vi "test Initial Label.vi"(8 "error in (no error)":errorcluster, 11 "TestCase in":refnum<class "Monitor Test.lvclass">) -> (0 "error out":errorcluster, 3 "TestCase out":refnum<class "Monitor Test.lvclass">)   [LabVIEW 2017, in "Monitor Test.lvclass"]
uses:
  Monitor Test.lvclass
  Source/Monitor Data/Actor Data.ctl
  <vilib>/ActorFramework/Message Enqueuer/Message Enqueuer.lvclass
  Test Actor/Test Actor.lvclass
  C:/Program Files (x86)/National Instruments/LabVIEW 2017/vi.lib/ActorFramework/Actor/Actor.lvclass
  <vilib>/ActorFramework/Message Enqueuer/Message Enqueuer.lvclass/Message Enqueuer.ctl
  <vilib>/ActorFramework/Message Enqueuer/Enqueue.vi
  <vilib>/ActorFramework/Stop Msg/Stop Msg.lvclass
  C:/Program Files (x86)/National Instruments/LabVIEW 2017/vi.lib/ActorFramework/Message/Message.lvclass
  <vilib>/ActorFramework/Message Priority Queue/Priority Enqueue.vi
  <vilib>/ActorFramework/Actor/Actor.lvclass
  Debug Monitor/Debug Monitor.lvclass
  Source/Monitor Data/Monitor Data.lvclass
panel:
  out "Actor Data":T1={"Actor Type"="", "Actor Cores"=[], "Self"=refnum, "Caller"=refnum, "Actor Label"="", "Last Ping"=-1.0}
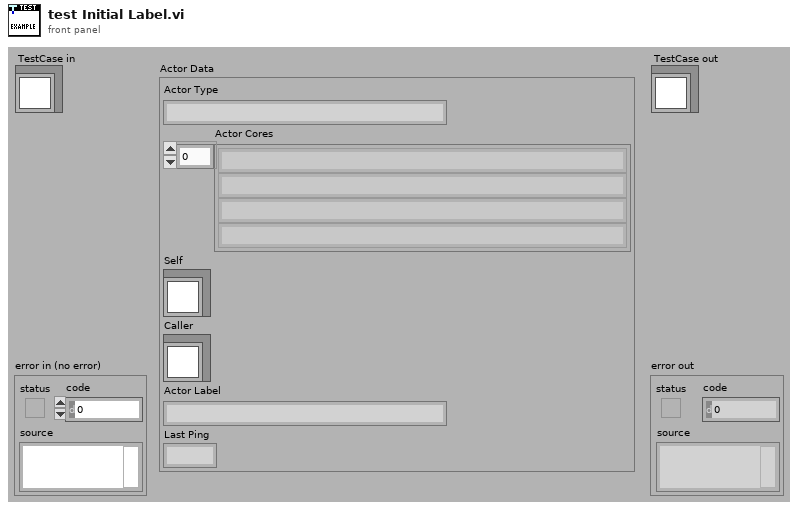
[diagram p1: front panel]
types:
  T1 = typedef "MGI-Monitored Actor Core.lvlib/Monitor Data.lvclass/Actor Data.ctl" = cluster{"Actor Type":string, "Actor Cores":string[], "Self":refnum<class "Message Enqueuer.lvclass">, "Caller":refnum<class "Message Enqueuer.lvclass">, "Actor Label":string, "Last Ping":dbl}
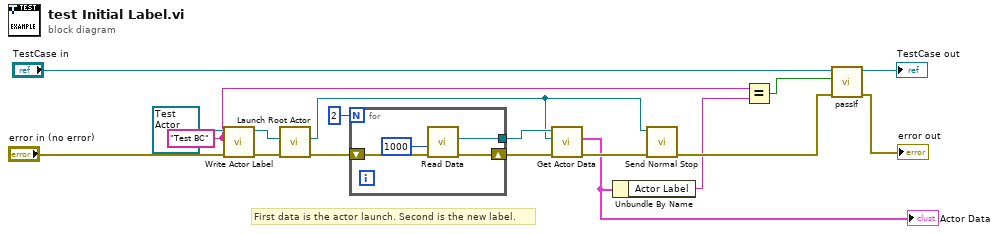
[diagram p0: block diagram]
diagram:
  w2 = "Test BC" ("Actor Label")
  # "First data is the actor launch. Second is the new label."
  n1 = call-dynamic "Write Actor Label.vi"("error in (no error)"="error in (no error)", "Actor Label"=w2, "Monitored Actor in"=refnum<class "Test Actor.lvclass"> refnum ("Test Actor.lvclass")) -> ("error out"=w5:errorcluster, "Monitored Actor out"=w7:refnum<class "Test Actor.lvclass">)  [unwired: 7 in]
  n2 = call <vilib>:"Launch Root Actor.vi"("error in (no error)"=w5, "Actor"=w7) -> ("error out"=w18:errorcluster, "Actor's Enqueuer"=w14:refnum<class "Message Enqueuer.lvclass">)  [unwired: 8 in]
  n3 = for {
    N: 2 -> [_]
    tunnel: [w20] -> w16
    shift-right: [w19] -> w15
    shift-left: w18 -> [w22]
    n4 = call "Read Data.vi"("error in (no error)"=w22, "timeout in ms (-1)"=1000) -> ("error out"=w19:errorcluster, "Monitor Data"=w20:refnum<class "Monitor Data.lvclass">)  [unwired: 7 in, 1 out]
  }
  n5 = call "Get Actor Data.vi"("error in (no error)"=w15, "Actor's Self Q"=w14, "Monitor Data in"=w16) -> ("error out"=w13:errorcluster, "Actor Data"=w8:T1)  [unwired: 5 in, 2 out]
  "Actor Data" <- w8
  n6 = Unbundle By Name(w8) -> ("Actor Label"=w4:string)
  n7 = call <vilib>:"Send Normal Stop.vi"("error in (no error)"=w13, "Message Enqueuer"=w14) -> ("error out"=w17:errorcluster)  [unwired: 9 in]
  n8 = Equal?(x=w2, y=w4) -> (x = y?=w3:bool)
  n9 = call-dynamic "passIf.vi"("error in (no error)"=w17, "pass"=w3, "TestCase in"="TestCase in") -> ("error out"=→"error out":errorcluster, "TestCase out"=→"TestCase out":refnum<class "Monitor Test.lvclass">)  [unwired: 7 in]
